vi "updateScanObj.vi"(2 "Scan Settings":T1={"A Scans"=300, "B Scans"=300, "Repeat B Scans"=1, "C Scans"=1.0, "X FOV (°)"=10.0, "Y FOV (°)"=10.0, "Rotate Scan (°)"=0.0, "X Offset (°)"=0.0, "Y Offset (°)"=0.0, "Bidirectional\nScanning"=FALSE, "Raster Type"="Rectangle", "Angio Mode"="None"} {"Y FOV (°)" min=0.0 step=0.5; "Repeat B Scans" min=1 step=1; "C Scans" min=1.0 step=1.0; "B Scans" min=1 step=1; "A Scans" min=100 max=1000 step=5; "Rotate Scan (°)" min=0.0 max=360.0 step=90.0; "X FOV (°)" min=0.0 step=0.5}, 3 "Scan in":refnum<class "Scan.lvclass">) -> (1 "Scan out":refnum<class "Scan.lvclass">)   [LabVIEW 2017]
uses:
  classes/Scans/Scan.lvclass
  classes/Scans/Scan.lvclass/Scan.ctl
  classes/Scans/Write A scans.vi
  classes/Scans/Write B scans.vi
  classes/Scans/Write C scans.vi
  classes/Scans/Write Repeat B scans.vi
  classes/Scans/Write Scan Angle (degrees).vi
  classes/Scans/Write Scan Pattern.vi
  classes/Scans/Write X FOV (degrees).vi
  classes/Scans/Write X offset (degrees).vi
  classes/Scans/Write Y FOV (degrees).vi
  classes/Scans/Write Y offset (degrees).vi
  classes/Scans/Write Bidirectional.vi
  classes/Scans/Write Angio Mode.vi
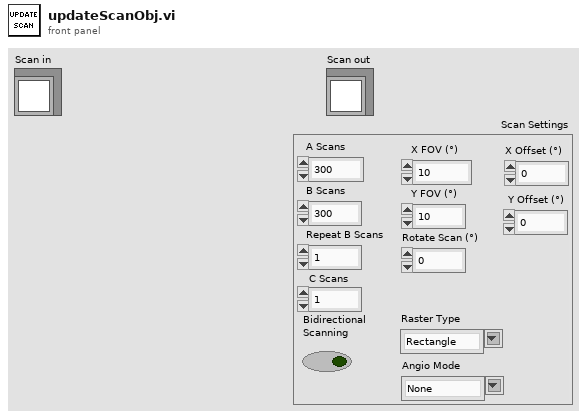
[diagram p1: front panel]
types:
  T1 = cluster{"A Scans":u32, "B Scans":u32, "Repeat B Scans":u32, "C Scans":dbl, "X FOV (°)":dbl, "Y FOV (°)":dbl, "Rotate Scan (°)":dbl, "X Offset (°)":dbl, "Y Offset (°)":dbl, "Bidirectional\nScanning":bool, "Raster Type":string, "Angio Mode":string}
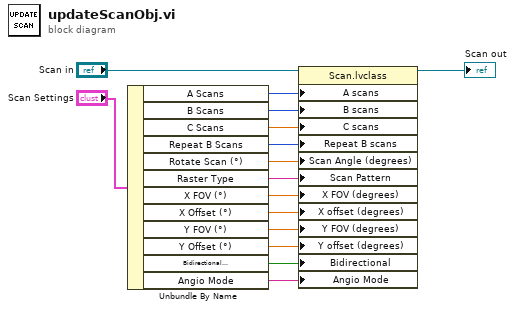
[diagram p0: block diagram]
diagram:
  n1 = Unbundle By Name("Scan Settings") -> ("A Scans"=w14:u32, "B Scans"=w13:u32, "C Scans"=w12:dbl, "Repeat B Scans"=w11:u32, "Rotate Scan (°)"=w10:dbl, "Raster Type"=w9:string, "X FOV (°)"=w8:dbl, "X Offset (°)"=w7:dbl, "Y FOV (°)"=w6:dbl, "Y Offset (°)"=w5:dbl, "Bidirectional\nScanning"=w4:bool, "Angio Mode"=w3:string)
  n2 = property class="Scan.lvclass"(reference="Scan in", "A scans"=w14, "B scans"=w13, "C scans"=w12, "Repeat B scans"=w11, "Scan Angle (degrees)"=w10, "Scan Pattern"=w9, "X FOV (degrees)"=w8, "X offset (degrees)"=w7, "Y FOV (degrees)"=w6, "Y offset (degrees)"=w5, "Bidirectional"=w4, "Angio Mode"=w3) -> (reference out=→"Scan out":refnum<class "Scan.lvclass">)  [unwired: 1 in, 1 out]
